vi "Modify Settings.vi"(6 "DV":dbl, 7 "M1 RF":dbl) -> (2 "DV 2":dbl, 3 "M1 RF 2":dbl)   [LabVIEW 2012]
panel:
  in  "Update":bool
  # "Please enter a new value for M1 RF and DV then press the update key."
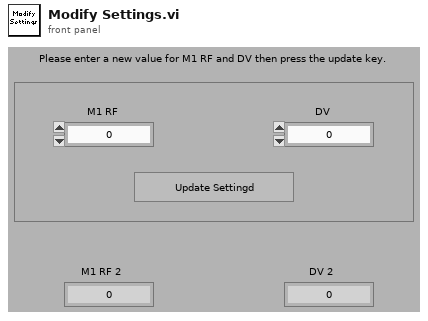
[diagram p1: front panel]
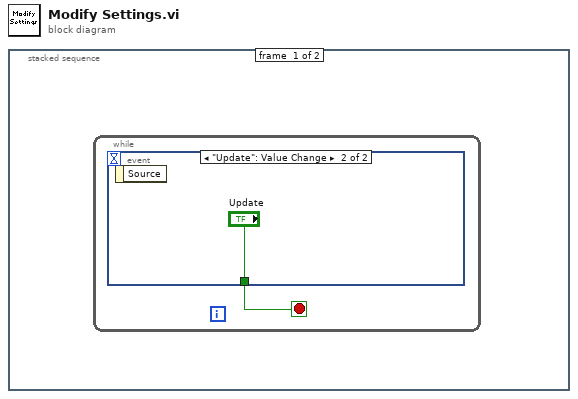
[diagram p0: block diagram]
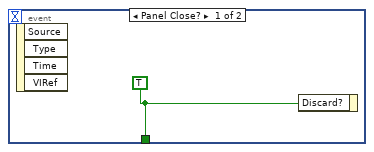
[diagram p2: hidden frame]
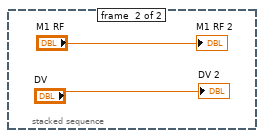
[diagram p3: hidden frame]
diagram:
  n1 = stacked-sequence {
    frame #0 {
      n2 = while {
        stop <- w1 stop-if-true
        n3 = event shown="[1] \"Update\": Value Change" {
          selector: _ -> [_ _]
          dyn-events: _ -> [_ _]
          timeout: _ -> [_ _]
          tunnel: [w2 "Update"] -> w1
          event Panel Close? {
            w2 = TRUE
            n4 = event-data() -> ()  [unwired: 5 out]
            n5 = event-data("Discard?"=w2) -> ()  [unwired: 1 in, 1 out]
          }
          event "Update": Value Change {
            n6 = event-data() -> ()  [unwired: 2 out]
          }
        }
      }
    }
    frame #1 {
      "DV 2" <- "DV"
      "M1 RF 2" <- "M1 RF"
    }
  }
